vi "0006 Path Management.vi"(7 "New?":bool, 8 "error in (no error)":errorcluster caption="Error In", 9 "Name":string, 10 "Path":T1, 11 "Path In":path) -> (0 "error out":errorcluster caption="Error Out", 2 "exists?":bool, 3 "Path Out":path)   [LabVIEW 2020]
uses:
  006 Path.ctl
  006 File Type.ctl
  006 System Gloabl.vi
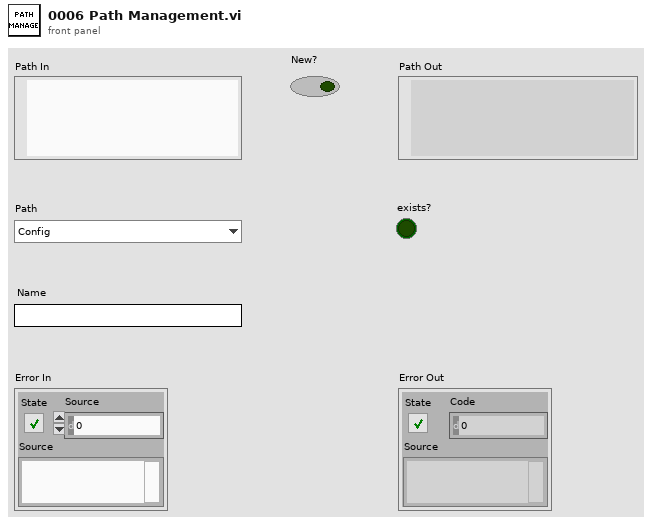
[diagram p1: front panel]
types:
  T1 = typedef "006 Path.ctl" = enum16{"Config", "Device.csv", "Version", "Project", "CertainProject", "Project Info.xml", "00_DataSource", "01_DataGraph", "02_DataSave", "03_TestProcess", "04_DataUse", "00_Database.mdb", "01_DataModule.xml", "02_ControlPanel.xml", "02_ControlPanelData.xml", "03_FlowChart.xml", "03_FlowChartData.xml", "04_Parameter_Setting.xml", "04_ParameterSettingData.xml"}
  T2 = typedef "006 File Type.ctl" = enum16{"Folder", "File"}
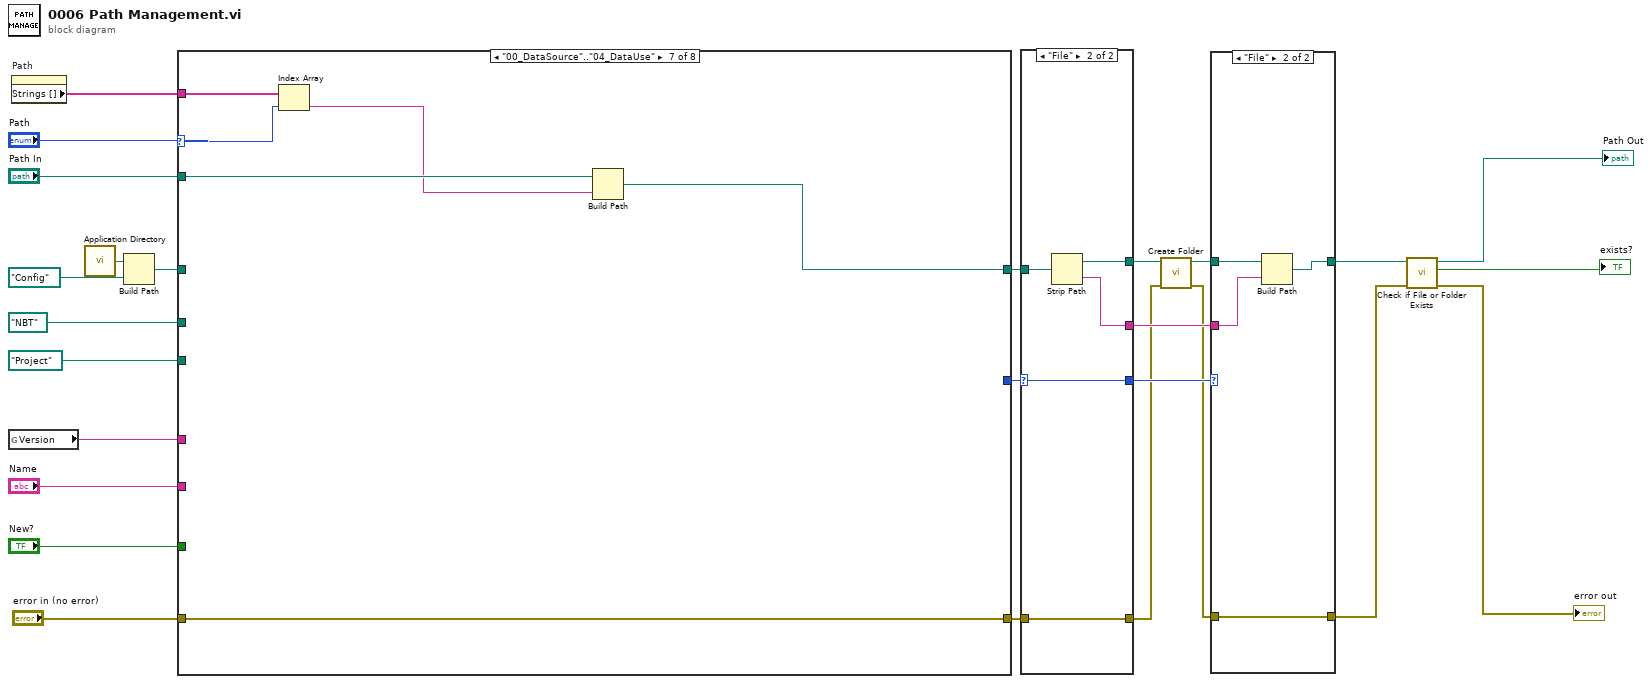
[diagram p0: block diagram]
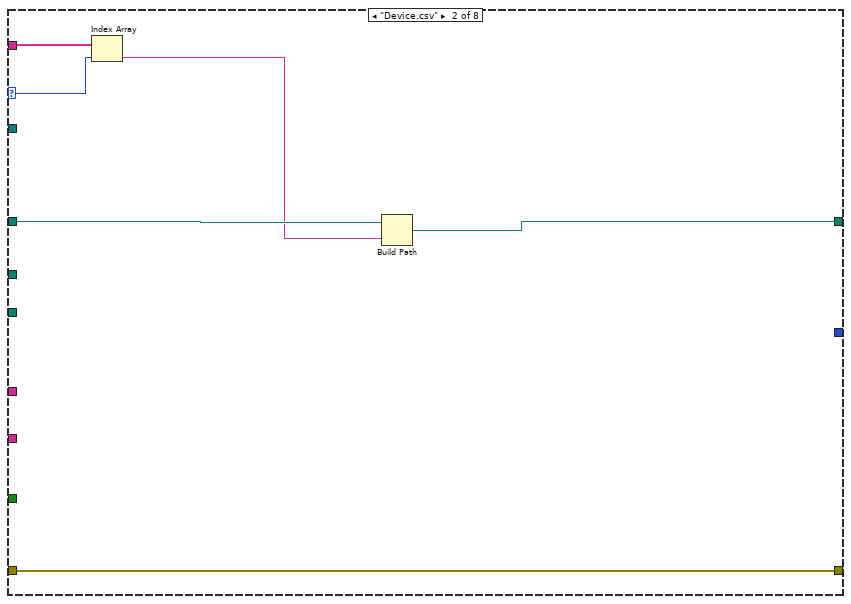
[diagram p4: hidden frame]
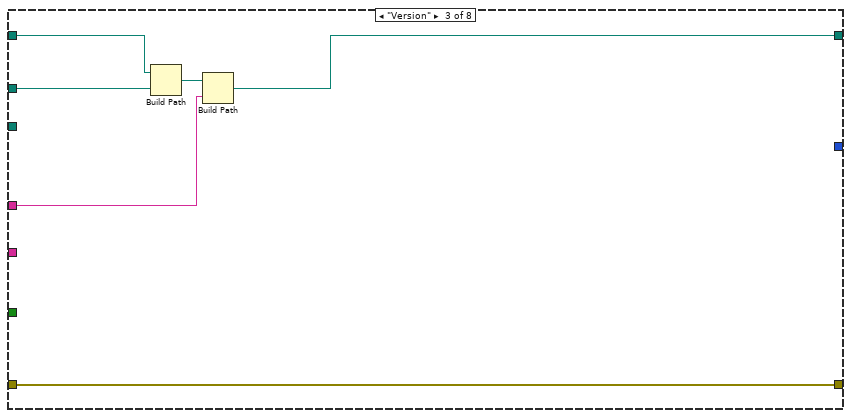
[diagram p5: hidden frame]
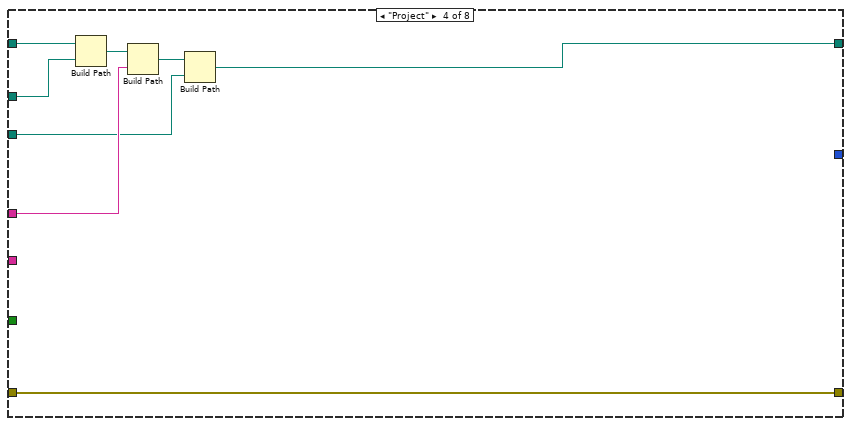
[diagram p6: hidden frame]
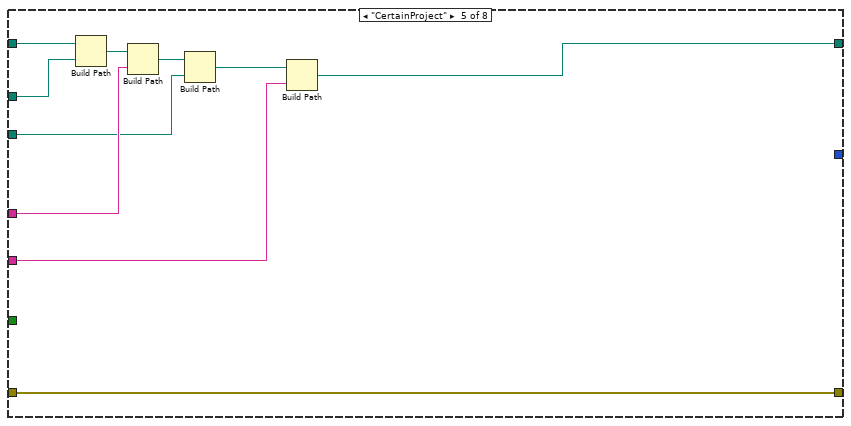
[diagram p7: hidden frame]
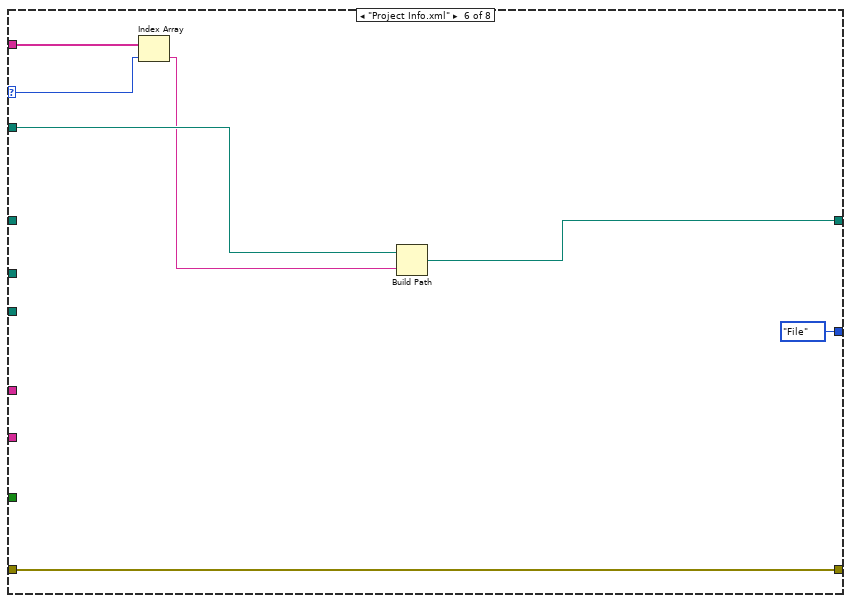
[diagram p8: hidden frame]
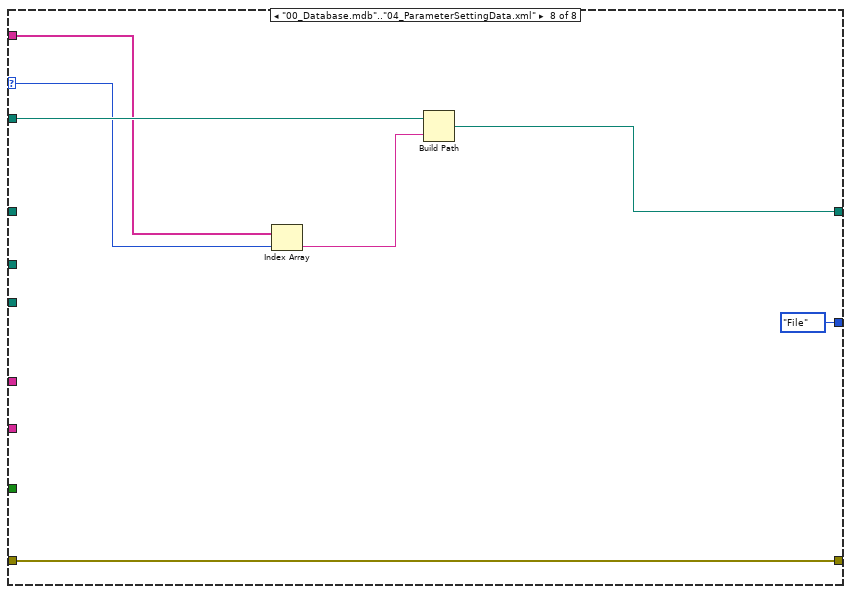
[diagram p9: hidden frame]
diagram:
  n1 = global read "006 System Gloabl.vi" "Version"() -> (w19:string)
  n2 = property on="Path" class="Enum (严格)"() -> ("Strings []"=w11:string[])  [unwired: 2 in, 2 out]
  n3 = call <vilib>:"Application Directory.vi"() -> ("Application Directory"=w26:path)
  n4 = Build Path(base path=w26, name or relative path=path "Config" ("名称或相对路径")) -> (appended path=w23:path)
  n5 = case shown="\"00_DataSource\"..\"04_DataUse\"" "Path" {
    selector: "Path" -> [_ w32 _ _ _ w62 w68 w75]
    tunnel: w23 -> [w28 w31 w39 w48 w58 _ _ _]
    tunnel: [_ _ _ _ _ 006_File_Type."File" ("Folder?") _ 006_File_Type."File" ("Folder?")] -> w22
    tunnel: [w28 w29 w36 w42 w49 w60 w70 w77] -> w21
    tunnel: path "NBT" ("名称或相对路径") -> [_ _ w38 w47 w57 _ _ _]
    tunnel: w19 -> [_ _ w37 w45 w55 _ _ _]
    tunnel: path "Project" ("名称或相对路径") -> [_ _ _ w43 w53 _ _ _]
    tunnel: "Name" -> [_ _ _ _ w50 _ _ _]
    tunnel: "New?" -> [_ _ _ _ _ _ _ _]
    tunnel: "Path In" -> [_ _ _ _ _ w63 w71 w78]
    tunnel: w11 -> [_ w33 _ _ _ w64 w69 w76]
    tunnel: "error in (no error)" -> [w27 w34 w35 w41 w52 w65 w66 w72]
    tunnel: [w27 w34 w35 w41 w52 w65 w66 w72] -> w7
    frame "Config", Default {
    }
    frame "Device.csv" {
      n6 = Index Array(array=w33, index=w32) -> (element=w30:string)
      n7 = Build Path(base path=w31, name or relative path=w30) -> (appended path=w29:path)
    }
    frame "Version" {
      n8 = Build Path(base path=w39, name or relative path=w38) -> (appended path=w40:path)
      n9 = Build Path(base path=w40, name or relative path=w37) -> (appended path=w36:path)
    }
    frame "Project" {
      n10 = Build Path(base path=w48, name or relative path=w47) -> (appended path=w46:path)
      n11 = Build Path(base path=w46, name or relative path=w45) -> (appended path=w44:path)
      n12 = Build Path(base path=w44, name or relative path=w43) -> (appended path=w42:path)
    }
    frame "CertainProject" {
      n13 = Build Path(base path=w58, name or relative path=w57) -> (appended path=w56:path)
      n14 = Build Path(base path=w56, name or relative path=w55) -> (appended path=w54:path)
      n15 = Build Path(base path=w54, name or relative path=w53) -> (appended path=w51:path)
      n16 = Build Path(base path=w51, name or relative path=w50) -> (appended path=w49:path)
    }
    frame "Project Info.xml" {
      n17 = Index Array(array=w64, index=w62) -> (element=w61:string)
      n18 = Build Path(base path=w63, name or relative path=w61) -> (appended path=w60:path)
    }
    frame "00_DataSource".."04_DataUse" {
      n19 = Index Array(array=w69, index=w68) -> (element=w67:string)
      n20 = Build Path(base path=w71, name or relative path=w67) -> (appended path=w70:path)
    }
    frame "00_Database.mdb".."04_ParameterSettingData.xml" {
      n21 = Index Array(array=w76, index=w75) -> (element=w74:string)
      n22 = Build Path(base path=w78, name or relative path=w74) -> (appended path=w77:path)
    }
  }
  n23 = case shown="\"File\"" w22 {
    selector: w22 -> [w80 w84]
    tunnel: w21 -> [w81 w86]
    tunnel: [w81 w85] -> w17
    tunnel: [w80 w84] -> w12
    tunnel: [_ w83] -> w10
    tunnel: [w79 w82] -> w8
    tunnel: w7 -> [w79 w82]
    frame "Folder", Default {
    }
    frame "File" {
      n24 = Strip Path(path=w86) -> (stripped path=w85:path, name=w83:string)
    }
  }
  n25 = call "Create Folder.vi"("error in (no error)"=w8, "Path In"=w17) -> ("error out"=w6:errorcluster, "Path Out"=w16:path)  [unwired: 8 in]
  n26 = case shown="\"File\"" w12 {
    tunnel: w16 -> [w88 w92]
    tunnel: [w88 w91] -> w5
    tunnel: w10 -> [_ w90]
    tunnel: w6 -> [w87 w89]
    tunnel: [w87 w89] -> w3
    frame "Folder", Default {
    }
    frame "File" {
      n27 = Build Path(base path=w92, name or relative path=w90) -> (appended path=w91:path)
    }
  }
  n28 = call <vilib>:"Check if File or Folder Exists.vi"("error in (no error)"=w3, "path"=w5) -> ("error out"=→"error out":errorcluster, "file or folder exists?"=→"exists?":bool, "dup path"=→"Path Out":path)  [unwired: 7 in]
